vi "Migrate Measurements.vi"() -> ()   [LabVIEW 2021]
uses:
  _Measurement Migrator/Migrator/Queue Driver/controls/Queue Operations.ctl
  _Measurement Migrator/Migrator/Migration Logic/controls/Multiple Migration/Multiple Migration Data Holder.ctl
  <vilib>/Utility/sysdir.llb/System Directory Type.ctl
  <vilib>/Utility/miscctls.llb/LVRowAndColumnUnsignedTypeDef.ctl
  <vilib>/Utility/miscctls.llb/LVRowAndColumnTypeDef.ctl
  _Measurement Migrator/Migrator/Migrator Reusables/controls/Dictionary States.ctl
  <vilib>/Utility/cursorutil.llb/Set Cursor (Icon Pict).vi
  _Measurement Migrator/Migrator/Queue Driver/Queue Driver.lvlib
  _Measurement Migrator/Migrator/Migration Logic/Migrator.lvlib
  _Measurement Migrator/Migrator/Path Functions/Path Functions.lvlib
  _Measurement Migrator/Migrator/Multiple Migrator/Multiple Migrator.lvlib
  _Measurement Migrator/Migrator/Migrator Reusables/Migrator Reusables.lvlib
panel:
  out "error out":errorcluster
  in  "Tab Control":T1(tab)
  in  "Info":string
  in  "Select Measurement":path
  out "Warning":bool=TRUE caption="Warning:\nMeasurement should be an existing VI or folder path"
  in  "Populate measurements":bool
  in  "Select Project":path
  in  "Select all":bool
  in  "Back to Home":bool
  in  "List Plug-ins":bool
  in  "Select Measurements":string(tree)
  out "Selection warning":string="Atleast one measurement should be selected"
  out "Plug-in info":string="* Rename the Plug-in if required"
  out "Plug-in warning":string="Warning:\n1. Measurement plug-in name must be unique \n2. Plugin name cannot contain any of the following characters:\n         \\ / : * ? \" < > |"
  in  "Start Migration":bool
  in  "Back to Select":bool
  in  "List of Selected Measurements":i32(listbox)
  in  "Measurement Count":i32(slide)=6 caption="Migrating 1 of 1 measurement(s)" scale=0.0..100.0
  in  "Progress":i32(slide)=9 caption="Saving the project files..." scale=0.0..15.0
  in  "Review":bool
  in  "Migration Status":i32(listbox)
  in  "Back to Status":bool
  in  "Select Plug-in":string(combo) caption="Select Measurement plug-in to review"
  in  "Start Next":bool
  out "Launch Type Spec":string
  out "Launch Logic":string
  out "Launch UI":string
  # "* Project in which the measurement plug-in will be created"
  # "* Select a measurement vi or a folder containing measurements"
  # ".lvproj"
  # "Select the measurements to migrate"
  # "Review the Measurement:\n1. Review the Measurement UI. Click here to launch.\n2. Review the Measurement Logic VI. Click here to launch.\n3. Review the Type Specialization VI. Click here to launch."
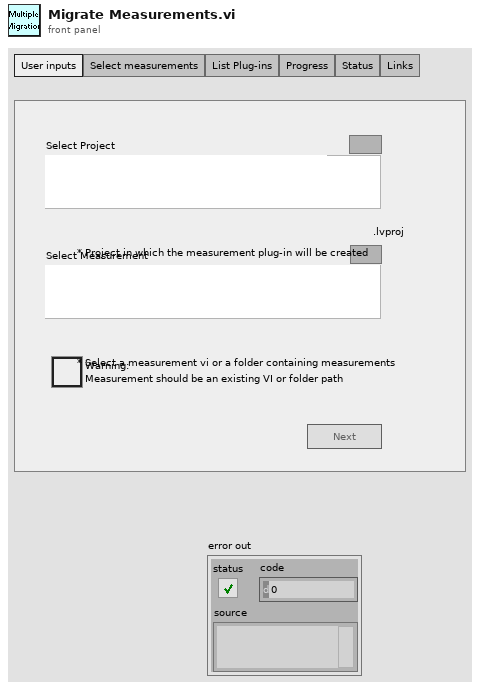
[diagram p1: front panel]
types:
  T1 = enum32{"User inputs", "Select measurements", "List Plug-ins", "Progress", "Status", "Links"}
  T2 = typedef "Queue Driver.lvlib/Queue Operations.ctl" = enum16{"Create Q", "Enqueue", "Enqueue N", "Dequeue", "Flush", "Release"}
  T3 = typedef "Migrator.lvlib/Multiple Migration Data Holder.ctl" = cluster{"Tree Reference":refnum<vi>, "LabVIEW Version":string, "Project path":path, "Create new project?":bool, "Measurement file/folder path":path, "Measurement folder selected?":bool, "Project warning":string, "Measurement warning":string, "Next clicked?":bool, "Measurement path changed?":bool, "Select all":bool, "Measurement folder Tags":string[], "Measurement file Tags":string[], "Selected cell Tag":string, "Measurement Plug-ins":string[][], "Measurement File Paths":path[], "Plugin Migration Value":i32, "Migration Count":i32, "Instrument containing subVIs":path[][], "Progress per measurement":i32, "Measurement Progress":i32, "Migration Status":string[][]}
  T4 = enum8{"Enabled", "Disabled", "Disabled and Grayed Out"}
  T5 = typedef "LVRowAndColumnUnsignedTypeDef.ctl" = cluster{"Row":u32, "Column":u32}
  T6 = typedef "LVRowAndColumnTypeDef.ctl" = cluster{"Row":i32, "Column":i32}
  T7 = typedef "Migrator Reusables.lvlib/Dictionary States.ctl" = enum16{"Set", "Get", "Delete", "Delete All"}
  T8 = typedef "System Directory Type.ctl" = i32
  T9 = typedef "LVPoint32TypeDef.ctl" = cluster{"Horizontal":i32, "Vertical":i32}
  T10 = typedef "Migrator.lvlib/Tree Items.ctl" = cluster{"Item name":string, "Indent":i32, "Tag":string}
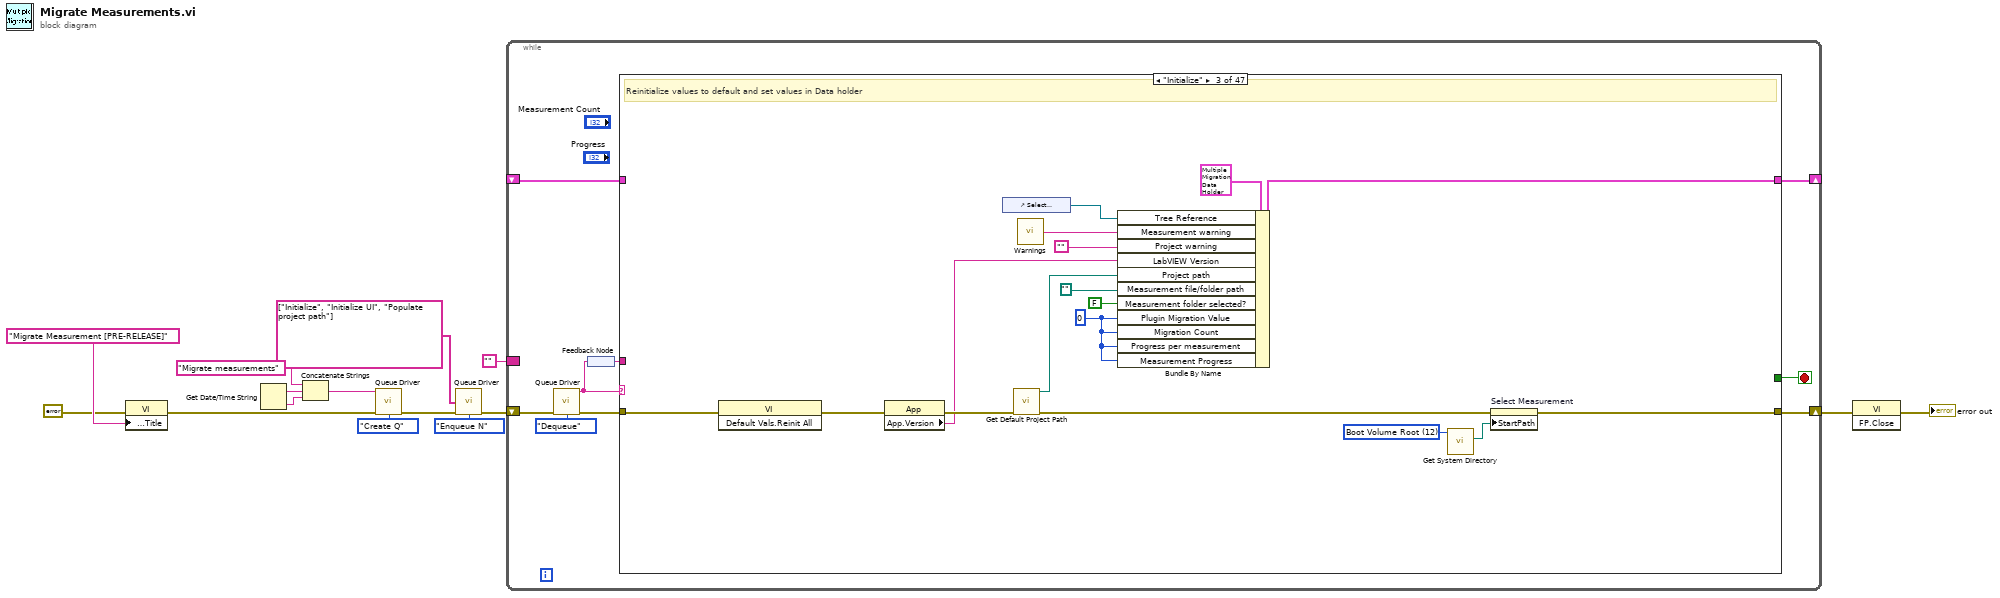
[diagram p0: block diagram]
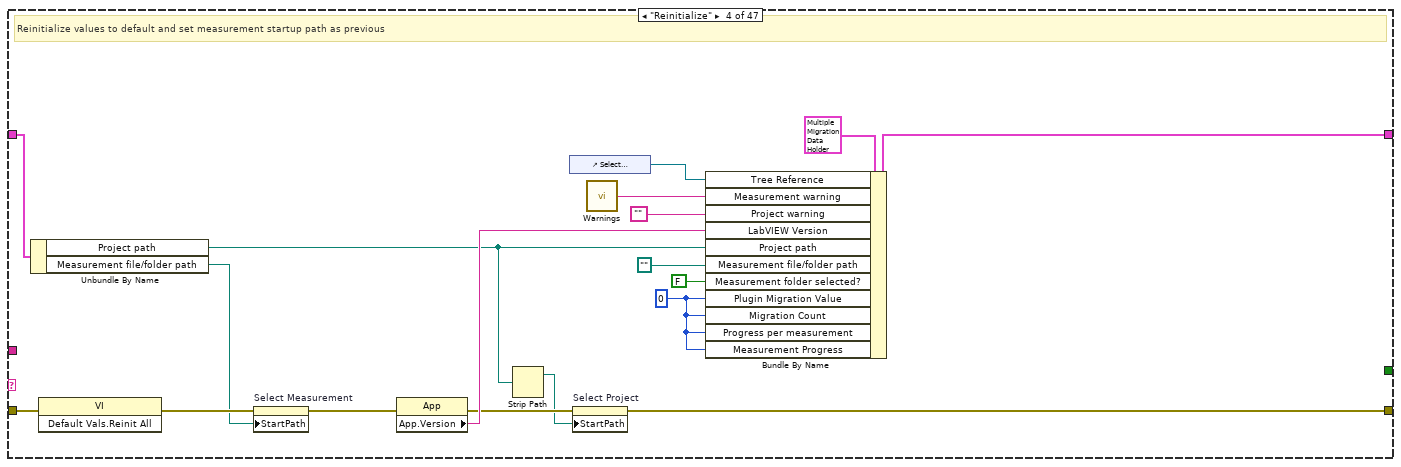
[diagram p4: hidden frame]
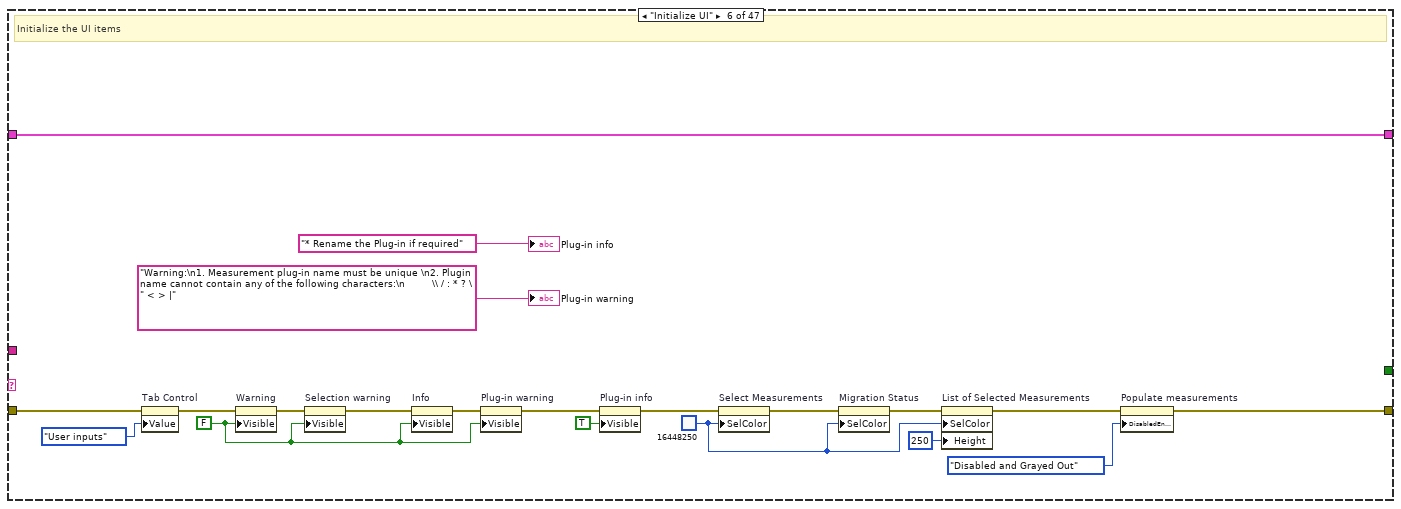
[diagram p6: hidden frame]
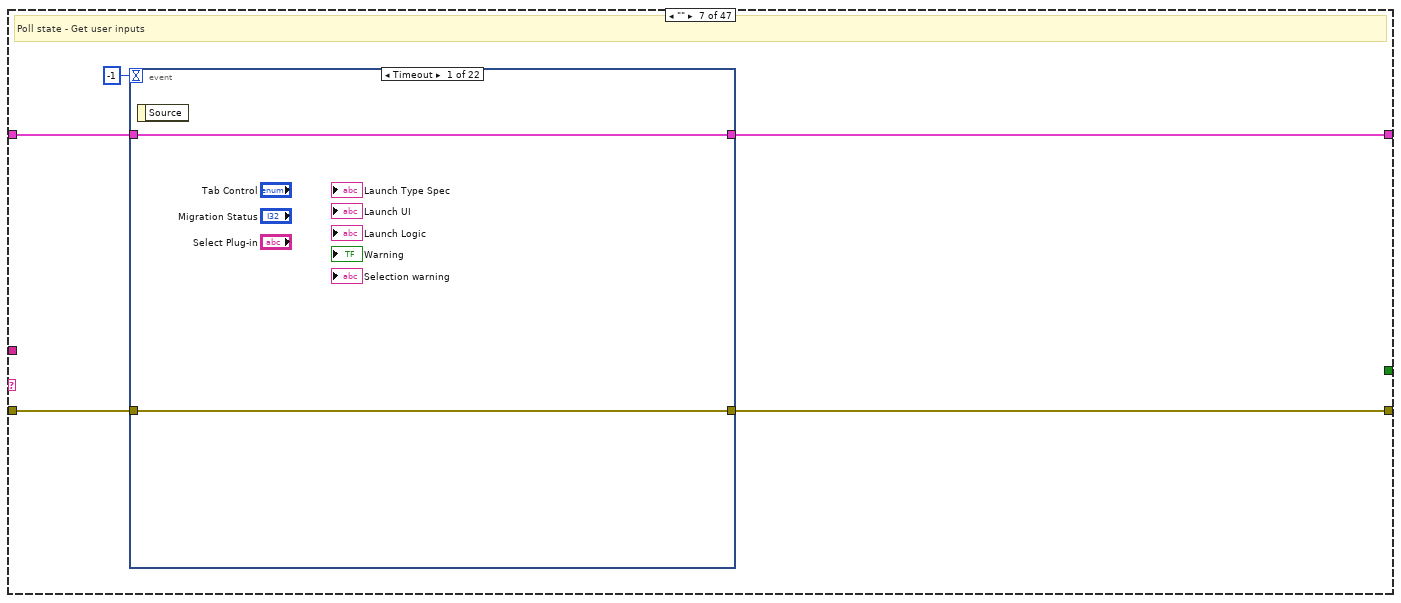
[diagram p7: hidden frame]
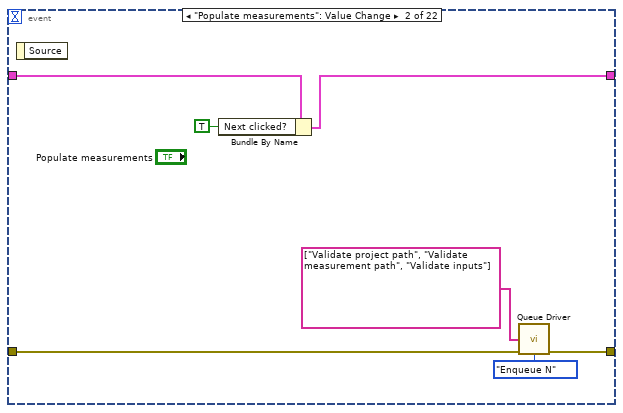
[diagram p8: hidden frame]
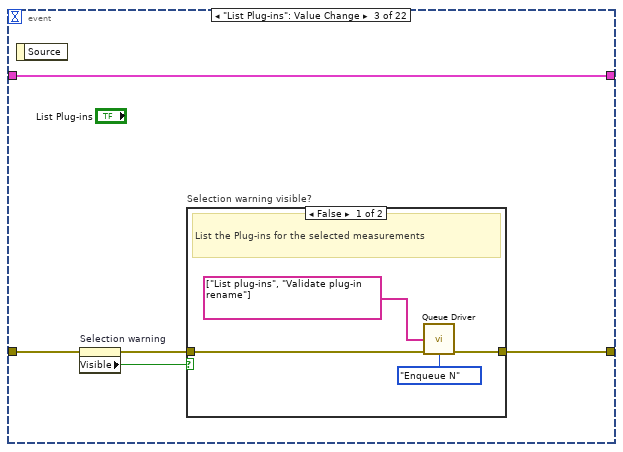
[diagram p9: hidden frame]
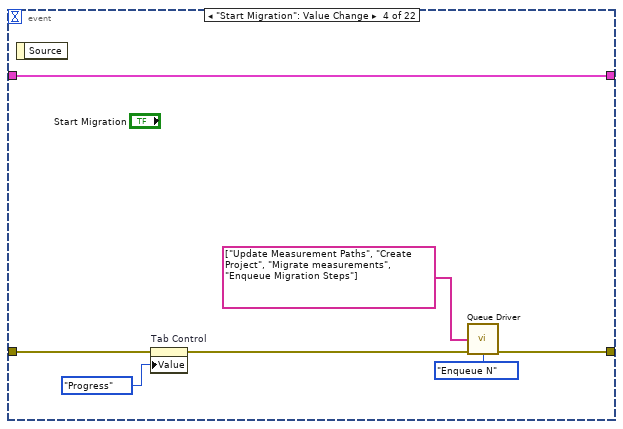
[diagram p11: hidden frame]
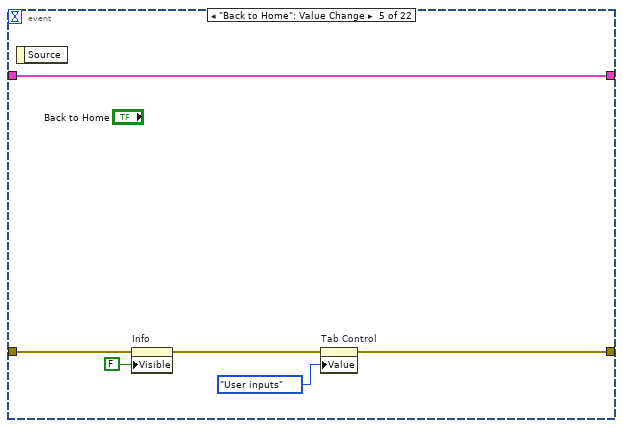
[diagram p12: hidden frame]
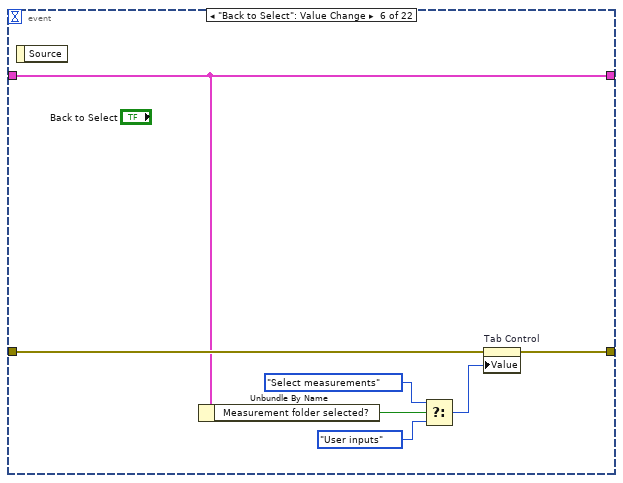
[diagram p13: hidden frame]
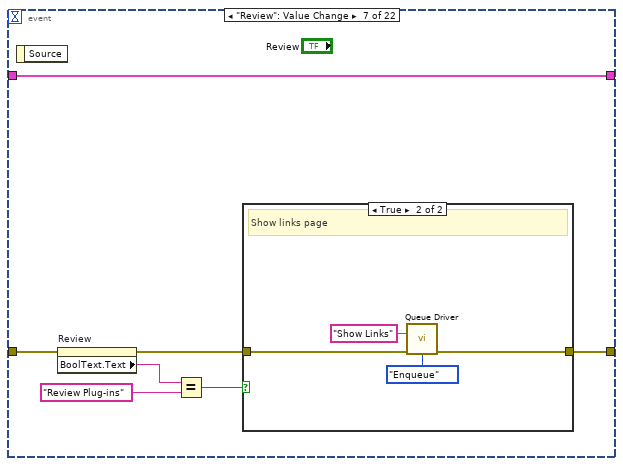
[diagram p14: hidden frame]
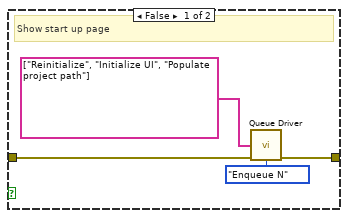
[diagram p15: hidden frame]
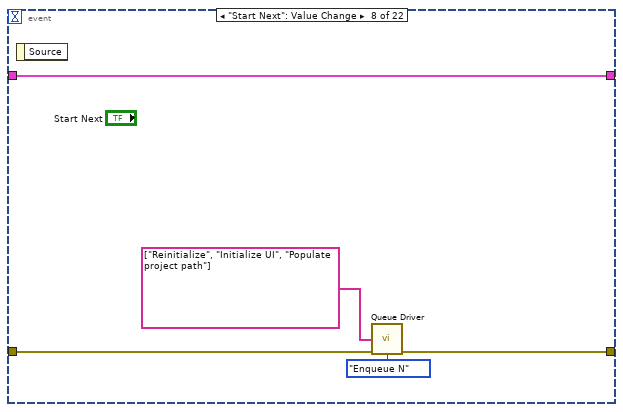
[diagram p16: hidden frame]
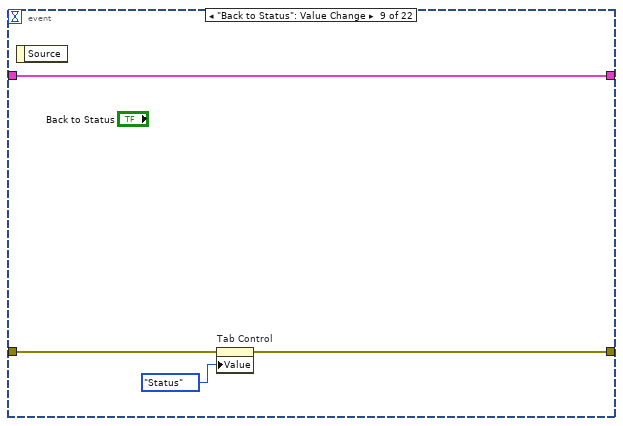
[diagram p17: hidden frame]
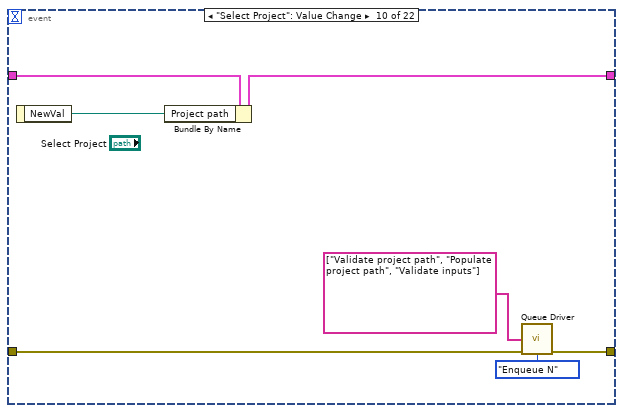
[diagram p18: hidden frame]
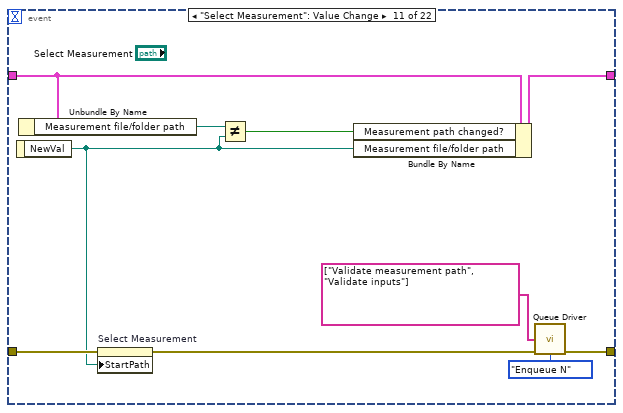
[diagram p19: hidden frame]
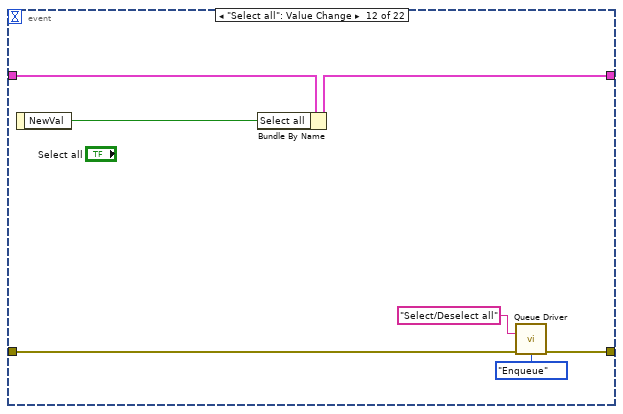
[diagram p20: hidden frame]
diagram:
  n1 = property class="VI"(error in=errorcluster {"status"=FALSE, "code"=0, "source"=""} ("error in (no error)"), "Front Panel.Title"="Migrate Measurement [PRE-RELEASE]" ("Front Panel Window:Title")) -> (error out=w1:errorcluster)  [unwired: 1 in, 1 out]
  n2 = Get Date/Time String() -> (date string=w12:string, time string=w11:string)  [unwired: 3 in]
  n3 = Concatenate Strings("Migrate measurements" ("string"), w12, w11) -> (w7:string)
  n4 = call "Queue Driver.vi"("Name"=w7, "error in (no error)"=w1, "Q Operations"=Queue_Operations."Create Q") -> ("error out"=w15:errorcluster)  [unwired: 11 in, 1 out]
  n5 = call "Queue Driver.vi"("States[]"=string[] ["Initialize", "Initialize UI", "Populate project path"], "error in (no error)"=w15, "Q Operations"=Queue_Operations."Enqueue N") -> ("error out"=w10:errorcluster)  [unwired: 11 in, 1 out]
  n6 = while {
    shift-right: [w23] -> w6
    shift-left: w10 -> [w24]
    shift-right: [w20] -> _
    shift-left: _ -> [w19]
    border: "" -> [_]
    stop <- w18 stop-if-true
    n7 = call "Queue Driver.vi"("error in (no error)"=w24, "Q Operations"=Queue_Operations."Dequeue") -> ("Dequeued State"=w17:string, "error out"=w22:errorcluster)  [unwired: 12 in]
    n8 = feedback #1() -> (w16:string)
    n9 = feedback-in #1(w17) -> ()
    n10 = case shown="\"Initialize\"" w17 {
      tunnel: w22 -> [w25 w28 w45 w63 w65 w85 w90 w262 w274 w285 w304 w328 w373 w390 w443 w468 w487 w544 w554 w560 w583 w593 w612 w629 w651 w658 w664 w670 w676 w682 w688 w694 w700 w706 w712 w718 w724 w730 w736 w758 w779 w791 w833 w842 w851 w872 w884]
      tunnel: [w25 w28 w34 w48 w65 w76 w89 w264 w274 w277 w303 w327 w373 w385 w431 w451 w474 w534 w554 w555 w580 w596 w611 w628 w650 w660 w666 w672 w678 w684 w690 w696 w702 w708 w714 w720 w726 w731 w740 w762 w779 w790 w830 w842 w848 w872 w874] -> w23
      tunnel: [w26 w27 w44 w62 w64 w81 w86 w263 w275 w280 w297 w315 w374 w391 w434 w466 w471 w539 w553 w575 w591 w605 w615 w648 w656 w662 w668 w674 w680 w686 w692 w698 w704 w710 w716 w722 w728 w734 w741 w763 w780 w795 w832 w843 w853 w873 w882] -> w20
      tunnel: w19 -> [w26 w27 _ w51 w64 w81 w87 w263 w275 w281 w299 w326 w374 w392 w435 w467 w472 w540 w553 w576 w591 w604 w615 w648 w656 w662 w668 w674 w680 w686 w692 w698 w704 w710 w716 w722 w728 w734 w742 w764 w780 w796 w832 w843 w853 w873 w882]
      tunnel: [_ _ _ _ _ _ _ _ _ _ _ _ _ _ _ _ _ _ _ _ _ _ _ _ _ _ _ _ _ _ _ _ _ _ _ _ _ _ _ _ _ _ _ _ _ _ TRUE] -> w18
      tunnel: w16 -> [_ _ _ _ _ _ _ _ _ _ _ _ _ _ _ _ _ _ _ _ _ _ _ _ _ _ _ _ _ _ _ _ _ _ _ _ _ _ _ _ _ _ _ _ w844 _ _]
      frame Default {
        # "Default case"
      }
      frame "/**********INITIALIZE**********/" {
      }
      frame "Initialize" {
        w29 = 0 ("Plugin Migration Value")
        w33 = T8 12 items=["User Home"=0, "User Desktop"=1, "User Documents"=2, "User Application Data"=3, "User Preferences"=4, "User Temporary"=5, "Public Documents"=6, "Public Application Data"=7, "Public Preferences"=8, "Public Cache"=13, "System Core Libraries"=9, "System Installed Libraries"=10, "Application Files"=11, "Boot Volume Root"=12] ("system directory type")
        # "Reinitialize values to default and set values in Data holder"
        n11 = invoke class="VI" method="Default Vals.Reinit All"(error in=w45) -> (error out=w42:errorcluster)  [unwired: 2 in, 2 out]
        n12 = property class="App"(error in=w42) -> (error out=w41:errorcluster, "App.Version"=w40:string)  [unwired: 1 in, 1 out]
        n13 = control-ref of="Select Measurements"() -> (w37:refnum<vi>)
        n14 = call "Get Default Project Path.vi"("error in"=w41) -> ("Project Path"=w43:path, "error out"=w35:errorcluster)  [unwired: 13 in]
        n15 = call "Warnings.vi"() -> ("Invalid measurement path"=w36:string)  [unwired: 8 in, 7 out]
        n16 = Bundle By Name(cluster=T3 {"Tree Reference"=refnum, "LabVIEW Version"="", "Project path"=path "", "Create new project?"=FALSE, "Measurement file/folder path"=path "", "Measurement folder selected?"=FALSE, "Project warning"="", "Measurement warning"="", "Next clicked?"=FALSE, "Measurement path changed?"=FALSE, "Select all"=FALSE, "Measurement folder Tags"=[], "Measurement file Tags"=[], "Selected cell Tag"="", "Measurement Plug-ins"=[], "Measurement File Paths"=[], "Plugin Migration Value"=0, "Migration Count"=0, "Instrument containing subVIs"=[], "Progress per measurement"=0, "Measurement Progress"=0, "Migration Status"=[]}, "Tree Reference"=w37, "Measurement warning"=w36, "Project warning"="", "LabVIEW Version"=w40, "Project path"=w43, "Measurement file/folder path"=path "", "Measurement folder selected?"=FALSE, "Plugin Migration Value"=w29, "Migration Count"=w29, "Progress per measurement"=w29, "Measurement Progress"=w29) -> (w44:T3)
        n17 = call <vilib>:"Get System Directory.vi"("system directory type"=w33) -> ("system directory"=w32:path)  [unwired: 10 in]
        n18 = property on="Select Measurement" class="Path"(error in=w35, "StartPath"=w32) -> (error out=w34:errorcluster)  [unwired: 1 in, 1 out]
      }
      frame "Reinitialize" {
        w54 = 0 ("Plugin Migration Value")
        # "Reinitialize values to default and set measurement startup path as previous"
        n19 = Unbundle By Name(w51) -> ("Project path"=w47:path, "Measurement file/folder path"=w50:path)
        n20 = invoke class="VI" method="Default Vals.Reinit All"(error in=w63) -> (error out=w53:errorcluster)  [unwired: 2 in, 2 out]
        n21 = property on="Select Measurement" class="Path"(error in=w53, "StartPath"=w50) -> (error out=w52:errorcluster)  [unwired: 1 in, 1 out]
        n22 = property class="App"(error in=w52) -> (error out=w49:errorcluster, "App.Version"=w61:string)  [unwired: 1 in, 1 out]
        n23 = Strip Path(path=w47) -> (stripped path=w46:path)  [unwired: 1 out]
        n24 = control-ref of="Select Measurements"() -> (w58:refnum<vi>)
        n25 = property on="Select Project" class="Path"(error in=w49, "StartPath"=w46) -> (error out=w48:errorcluster)  [unwired: 1 in, 1 out]
        n26 = call "Warnings.vi"() -> ("Invalid measurement path"=w57:string)  [unwired: 8 in, 7 out]
        n27 = Bundle By Name(cluster=T3 {"Tree Reference"=refnum, "LabVIEW Version"="", "Project path"=path "", "Create new project?"=FALSE, "Measurement file/folder path"=path "", "Measurement folder selected?"=FALSE, "Project warning"="", "Measurement warning"="", "Next clicked?"=FALSE, "Measurement path changed?"=FALSE, "Select all"=FALSE, "Measurement folder Tags"=[], "Measurement file Tags"=[], "Selected cell Tag"="", "Measurement Plug-ins"=[], "Measurement File Paths"=[], "Plugin Migration Value"=0, "Migration Count"=0, "Instrument containing subVIs"=[], "Progress per measurement"=0, "Measurement Progress"=0, "Migration Status"=[]}, "Tree Reference"=w58, "Measurement warning"=w57, "Project warning"="", "LabVIEW Version"=w61, "Project path"=w47, "Measurement file/folder path"=path "", "Measurement folder selected?"=FALSE, "Plugin Migration Value"=w54, "Migration Count"=w54, "Progress per measurement"=w54, "Measurement Progress"=w54) -> (w62:T3)
      }
      frame "/**********FP RELATED**********/" {
      }
      frame "Initialize UI" {
        w70 = FALSE ("Visible")
        w78 = u32 16448250 ("Selection Color")
        # "Initialize the UI items"
        n28 = property on="Tab Control" class="TabCtl (strict)"(error in=w85, "Value"=T1."User inputs" ("Tab Control")) -> (error out=w80:errorcluster)  [unwired: 1 in, 1 out]
        n29 = property on="Warning" class="Bool"(error in=w80, "Visible"=w70) -> (error out=w79:errorcluster)  [unwired: 1 in, 1 out]
        n30 = property on="Selection warning" class="Str"(error in=w79, "Visible"=w70) -> (error out=w74:errorcluster)  [unwired: 1 in, 1 out]
        n31 = property on="Info" class="Str"(error in=w74, "Visible"=w70) -> (error out=w73:errorcluster)  [unwired: 1 in, 1 out]
        n32 = property on="Plug-in warning" class="Str"(error in=w73, "Visible"=w70) -> (error out=w69:errorcluster)  [unwired: 1 in, 1 out]
        n33 = property on="Plug-in info" class="Str"(error in=w69, "Visible"=TRUE) -> (error out=w68:errorcluster)  [unwired: 1 in, 1 out]
        n34 = property on="Select Measurements" class="Tree (strict)"(error in=w68, "SelColor"=w78) -> (error out=w83:errorcluster)  [unwired: 1 in, 1 out]
        n35 = property on="Migration Status" class="MCListbox (strict)"(error in=w83, "SelColor"=w78) -> (error out=w82:errorcluster)  [unwired: 1 in, 1 out]
        n36 = property on="List of Selected Measurements" class="MCListbox (strict)"(error in=w82, "SelColor"=w78, "Height"=u32 250 ("Size:Height")) -> (error out=w77:errorcluster)  [unwired: 1 in, 1 out]
        n37 = property on="Populate measurements" class="Bool"(error in=w77, "DisabledEnum"=T4."Disabled and Grayed Out" ("Disabled")) -> (error out=w76:errorcluster)  [unwired: 1 in, 1 out]
        "Plug-in warning" <- "Warning:\n1. Measurement plug-in name must be unique \n2. Plugin name cannot contain any of the following characters:\n         \\ / : * ? \" < > |" ("f")
        "Plug-in info" <- "* Rename the Plug-in if required" ("Plug-in warning")
      }
      frame "" {
        # "Poll state - Get user inputs"
        n38 = event shown="[0] Timeout" {
          selector: _ -> [_ _ _ _ _ _ _ _ _ _ _ _ _ _ _ _ _ _ _ _ _ _]
          dyn-events: _ -> [_ _ _ _ _ _ _ _ _ _ _ _ _ _ _ _ _ _ _ _ _ _]
          timeout: -1 -> [_ _ _ _ _ _ _ _ _ _ _ _ _ _ _ _ _ _ _ _ _ _]
          tunnel: w90 -> [w92 w99 w102 w116 w119 w129 w133 w146 w153 w160 w166 w174 w185 w194 w202 w209 w212 w216 w222 w232 w244 w256]
          tunnel: [w92 w98 w103 w112 w122 w128 w135 w147 w152 w159 w169 w173 w180 w193 w200 w210 w213 w217 w224 w235 w246 w255] -> w89
          tunnel: w87 -> [w91 w95 w104 w113 w120 w127 w136 w149 w150 w157 w164 w177 w184 w195 w203 w211 w215 w219 w225 w236 w247 w257]
          tunnel: [w91 w94 w104 w113 w120 w127 w136 w149 w150 w156 w170 w176 w183 w195 w203 w211 w215 w219 w225 w236 w247 w257] -> w86
          event Timeout {
            # "Timeout"
            n39 = event-data() -> ()  [unwired: 1 in, 1 out]
          }
          event "Populate measurements": Value Change {
            n40 = event-data() -> ()  [unwired: 1 in, 1 out]
            n41 = Bundle By Name(cluster=w95, "Next clicked?"=TRUE) -> (w94:T3)
            n42 = call "Queue Driver.vi"("States[]"=string[] ["Validate project path", "Validate measurement path", "Validate inputs"], "error in (no error)"=w99, "Q Operations"=Queue_Operations."Enqueue N") -> ("error out"=w98:errorcluster)  [unwired: 11 in, 1 out]
          }
          event "List Plug-ins": Value Change {
            n43 = event-data() -> ()  [unwired: 1 in, 1 out]
            n44 = property on="Selection warning" class="Str"(error in=w102) -> (error out=w101:errorcluster, "Visible"=w100:bool)  [unwired: 1 in, 1 out]
            n45 = case "Selection warning visible?" shown="False" w100 {
              tunnel: w101 -> [w108 w109]
              tunnel: [w107 w109] -> w103
              frame False {
                # "List the Plug-ins for the selected measurements"
                n46 = call "Queue Driver.vi"("States[]"=string[] ["List plug-ins", "Validate plug-in rename"], "error in (no error)"=w108, "Q Operations"=Queue_Operations."Enqueue N") -> ("error out"=w107:errorcluster)  [unwired: 11 in, 1 out]
              }
              frame True {
                # "Pass"
              }
            }
          }
          event "Start Migration": Value Change {
            n47 = event-data() -> ()  [unwired: 1 in, 1 out]
            n48 = property on="Tab Control" class="TabCtl (strict)"(error in=w116, "Value"=T1."Progress" ("Tab Control")) -> (error out=w115:errorcluster)  [unwired: 1 in, 1 out]
            n49 = call "Queue Driver.vi"("States[]"=string[] ["Update Measurement Paths", "Create Project", "Migrate measurements", "Enqueue Migration Steps"], "error in (no error)"=w115, "Q Operations"=Queue_Operations."Enqueue N") -> ("error out"=w112:errorcluster)  [unwired: 11 in, 1 out]
          }
          event "Back to Home": Value Change {
            n50 = event-data() -> ()  [unwired: 1 in, 1 out]
            n51 = property on="Info" class="Str"(error in=w119, "Visible"=FALSE) -> (error out=w118:errorcluster)  [unwired: 1 in, 1 out]
            n52 = property on="Tab Control" class="TabCtl (strict)"(error in=w118, "Value"=T1."User inputs" ("Tab Control")) -> (error out=w122:errorcluster)  [unwired: 1 in, 1 out]
          }
          event "Back to Select": Value Change {
            n53 = event-data() -> ()  [unwired: 1 in, 1 out]
            n54 = Unbundle By Name(w127) -> ("Measurement folder selected?"=w126:bool)
            n55 = Select(t=T1."Select measurements" ("Tab Control"), s=w126, f=T1."User inputs" ("Tab Control")) -> (s? t:f=w123:T1)
            n56 = property on="Tab Control" class="TabCtl (strict)"(error in=w129, "Value"=w123) -> (error out=w128:errorcluster)  [unwired: 1 in, 1 out]
          }
          event "Review": Value Change {
            n57 = event-data() -> ()  [unwired: 1 in, 1 out]
            n58 = property on="Review" class="Bool"(error in=w133) -> (error out=w134:errorcluster, "BoolText.Text"=w132:string)  [unwired: 1 in, 1 out]
            n59 = Equal?(x=w132, y="Review Plug-ins") -> (x = y?=w130:bool)
            n60 = case shown="True" w130 {
              tunnel: [w138 w144] -> w135
              tunnel: w134 -> [w137 w141]
              frame False {
                # "Show start up page"
                n61 = call "Queue Driver.vi"("States[]"=string[] ["Reinitialize", "Initialize UI", "Populate project path"], "error in (no error)"=w137, "Q Operations"=Queue_Operations."Enqueue N") -> ("error out"=w138:errorcluster)  [unwired: 11 in, 1 out]
              }
              frame True {
                # "Show links page"
                n62 = call "Queue Driver.vi"("State"="Show Links", "error in (no error)"=w141, "Q Operations"=Queue_Operations."Enqueue") -> ("error out"=w144:errorcluster)  [unwired: 11 in, 1 out]
              }
            }
          }
          event "Start Next": Value Change {
            n63 = event-data() -> ()  [unwired: 1 in, 1 out]
            n64 = call "Queue Driver.vi"("States[]"=string[] ["Reinitialize", "Initialize UI", "Populate project path"], "error in (no error)"=w146, "Q Operations"=Queue_Operations."Enqueue N") -> ("error out"=w147:errorcluster)  [unwired: 11 in, 1 out]
          }
          event "Back to Status": Value Change {
            n65 = event-data() -> ()  [unwired: 1 in, 1 out]
            n66 = property on="Tab Control" class="TabCtl (strict)"(error in=w153, "Value"=T1."Status" ("Tab Control")) -> (error out=w152:errorcluster)  [unwired: 1 in, 1 out]
          }
          event "Select Project": Value Change {
            n67 = event-data() -> ("NewVal"=w155:path)  [unwired: 1 in]
            n68 = Bundle By Name(cluster=w157, "Project path"=w155) -> (w156:T3)
            n69 = call "Queue Driver.vi"("States[]"=string[] ["Validate project path", "Populate project path", "Validate inputs"], "error in (no error)"=w160, "Q Operations"=Queue_Operations."Enqueue N") -> ("error out"=w159:errorcluster)  [unwired: 11 in, 1 out]
          }
          event "Select Measurement": Value Change {
            n70 = event-data() -> ("NewVal"=w161:path)  [unwired: 1 in]
            n71 = Unbundle By Name(w164) -> ("Measurement file/folder path"=w162:path)
            n72 = property on="Select Measurement" class="Path"(error in=w166, "StartPath"=w161) -> (error out=w165:errorcluster)  [unwired: 1 in, 1 out]
            n73 = Not Equal?(x=w162, y=w161) -> (x != y?=w163:bool)
            n74 = Bundle By Name(cluster=w164, "Measurement path changed?"=w163, "Measurement file/folder path"=w161) -> (w170:T3)
            n75 = call "Queue Driver.vi"("States[]"=string[] ["Validate measurement path", "Validate inputs"], "error in (no error)"=w165, "Q Operations"=Queue_Operations."Enqueue N") -> ("error out"=w169:errorcluster)  [unwired: 11 in, 1 out]
          }
          event "Select all": Value Change {
            n76 = event-data() -> ("NewVal"=w175:bool)  [unwired: 1 in]
            n77 = Bundle By Name(cluster=w177, "Select all"=w175) -> (w176:T3)
            n78 = call "Queue Driver.vi"("State"="Select/Deselect all", "error in (no error)"=w174, "Q Operations"=Queue_Operations."Enqueue") -> ("error out"=w173:errorcluster)  [unwired: 11 in, 1 out]
          }
          event "Select Measurements": Mouse Down {
            n79 = event-data() -> ("Coords"=w178:T9)  [unwired: 1 in]
            n80 = invoke on="Select Measurements" class="Tree (strict)" method="Point To Row Column"(error in=w185, "Point"=w178) -> (error out=w181:errorcluster, "Tag"=w182:string, "InGlyph"=w179:bool)  [unwired: 6 in, 5 out]
            n81 = case "In Symbol?" shown="True" w179 {
              tunnel: w181 -> [w186 w190]
              tunnel: [w186 w189] -> w180
              frame False {
                # "Pass"
              }
              frame True {
                # "Update the selection of measurements"
                n82 = call "Queue Driver.vi"("State"="Measurement selection" ("State 2"), "error in (no error)"=w190, "Q Operations"=Queue_Operations."Enqueue") -> ("error out"=w189:errorcluster)  [unwired: 11 in, 1 out]
              }
            }
            n83 = Bundle By Name(cluster=w184, "Selected cell Tag"=w182) -> (w183:T3)
          }
          event "List of Selected Measurements": Edit Cell {
            n84 = event-data() -> ()  [unwired: 1 in, 1 out]
            n85 = call "Queue Driver.vi"("State"="Validate plug-in rename", "error in (no error)"=w194, "Q Operations"=Queue_Operations."Enqueue") -> ("error out"=w193:errorcluster)  [unwired: 11 in, 1 out]
          }
          event "List of Selected Measurements": Mouse Down {
            n86 = event-data() -> ("Coords"=w199:T9)  [unwired: 1 in, 7 out]
            n87 = invoke on="List of Selected Measurements" class="MCListbox (strict)" method="Point To Row Column"(error in=w202, "Point"=w199) -> (error out=w201:errorcluster, "CellPosition"=w196:T6)  [unwired: 5 in, 5 out]
            n88 = Unbundle By Name(w196) -> ("Column"=w198:i32)
            n89 = Not Equal To 0?(x=w198) -> (x != 0?=w197:bool)
            n90 = case shown="False" w197 {
              tunnel: w201 -> [w204 w207]
              tunnel: [w204 w206] -> w200
              tunnel: w196 -> [_ w205]
              frame False {
              }
              frame True {
                n91 = property on="List of Selected Measurements" class="MCListbox (strict)"(error in=w207, "EditPos"=w205) -> (error out=w206:errorcluster)  [unwired: 1 in, 1 out]
              }
            }
          }
          event "Select Plug-in": Value Change {
            n92 = event-data() -> ("NewVal"=w208:string)  [unwired: 1 in]
            n93 = call "Set Measurement Name.vi"("Name"=w208, "error in (no error)"=w209) -> ("error out"=w210:errorcluster)  [unwired: 13 in]
          }
          event "Launch UI", "Launch Logic", "Launch Type Spec": Mouse Enter {
            n94 = event-data() -> ()  [unwired: 1 in, 1 out]
            n95 = call-poly <vilib>:"Set Cursor.vi"("error in (no error)"=w212, "icon"=u16 6) -> ("error out"=w213:errorcluster)  [unwired: 8 in, 1 out]
          }
          event "Launch UI", "Launch Logic", "Launch Type Spec": Mouse Leave {
            n96 = event-data() -> ()  [unwired: 1 in, 1 out]
            n97 = call-poly <vilib>:"Set Cursor.vi"("error in (no error)"=w216, "icon"=u16 0) -> ("error out"=w217:errorcluster)  [unwired: 8 in, 1 out]
          }
          event "Launch UI": Mouse Down {
            n98 = event-data() -> ()  [unwired: 1 in, 1 out]
            n99 = property on="Select Plug-in" class="CmbBox"(error in=w222) -> (error out=w223:errorcluster, "Value"=w221:string)  [unwired: 1 in, 1 out]
            n100 = Empty String/Path?(string/path=w221) -> (empty?=w220:bool)
            n101 = case shown="False" w220 {
              tunnel: [w228 w230] -> w224
              tunnel: w223 -> [w226 w230]
              frame False {
                n102 = call "Measurement Plugin Path.vi"("error in (no error)"=w226) -> ("Measurement UI"=w227:path, "error out"=w229:errorcluster)  [unwired: 2 in, 11 out]
                n103 = call "Open VI.vi"("Logic VI Path"=w227, "error in (no error)"=w229) -> ("error out"=w228:errorcluster)  [unwired: 13 in]
              }
              frame True {
              }
            }
          }
          event "Launch Logic": Mouse Down {
            n104 = event-data() -> ()  [unwired: 1 in, 1 out]
            n105 = property on="Select Plug-in" class="CmbBox"(error in=w232) -> (error out=w233:errorcluster, "Value"=w234:string)  [unwired: 1 in, 1 out]
            n106 = Empty String/Path?(string/path=w234) -> (empty?=w231:bool)
            n107 = case shown="False" w231 {
              tunnel: [w239 w241] -> w235
              tunnel: w233 -> [w238 w241]
              frame False {
                n108 = call "Measurement Plugin Path.vi"("error in (no error)"=w238) -> ("Logic VI Path"=w237:path, "error out"=w240:errorcluster)  [unwired: 2 in, 11 out]
                n109 = call "Open VI.vi"("Logic VI Path"=w237, "error in (no error)"=w240) -> ("error out"=w239:errorcluster)  [unwired: 13 in]
              }
              frame True {
              }
            }
          }
          event "Launch Type Spec": Mouse Down {
            n110 = event-data() -> ()  [unwired: 1 in, 1 out]
            n111 = property on="Select Plug-in" class="CmbBox"(error in=w244) -> (error out=w243:errorcluster, "Value"=w245:string)  [unwired: 1 in, 1 out]
            n112 = Empty String/Path?(string/path=w245) -> (empty?=w242:bool)
            n113 = case shown="False" w242 {
              tunnel: [w250 w252] -> w246
              tunnel: w243 -> [w249 w252]
              frame False {
                n114 = call "Measurement Plugin Path.vi"("error in (no error)"=w249) -> ("Type Specialization"=w248:path, "error out"=w251:errorcluster)  [unwired: 2 in, 11 out]
                n115 = call "Open VI.vi"("Logic VI Path"=w248, "error in (no error)"=w251) -> ("error out"=w250:errorcluster)  [unwired: 13 in]
              }
              frame True {
              }
            }
          }
          event Panel Close? {
            n116 = event-data() -> ()  [unwired: 1 in, 1 out]
            n117 = call "Queue Driver.vi"("State"="Exit", "error in (no error)"=w256, "Q Operations"=Queue_Operations."Enqueue") -> ("error out"=w255:errorcluster)  [unwired: 11 in, 1 out]
            n118 = event-data("Discard?"=TRUE) -> ()  [unwired: 1 in, 1 out]
          }
        }
      }
      frame "Populate project path" {
        # "Populate the validated project path in the control"
        n119 = Unbundle By Name(w263) -> ("Project warning"=w260:string, "Project path"=w261:path)
        n120 = Empty String/Path?(string/path=w260) -> (empty?=w259:bool)
        n121 = case "Valid project?" shown="True" w259 {
          tunnel: [w265 w273] -> w264
          tunnel: w262 -> [w265 w272]
          tunnel: w261 -> [_ w267]
          frame False {
            # "Pass"
          }
          frame True {
            # "Populate the path in the control"
            n122 = call <vilib>:"Get File Extension.vi"("error in (no error)"=w272, "file"=w267) -> ("error out"=w271:errorcluster, "filename without extension"=w270:string)  [unwired: 5 in, 3 out]
            n123 = Concatenate Strings("..\\" ("string"), w270) -> (w268:string)
            n124 = Build Path(base path=w267, name or relative path=w268) -> (appended path=w266:path)
            n125 = property on="Select Project" class="Path"(error in=w271, "Value"=w266) -> (error out=w273:errorcluster)  [unwired: 1 in, 1 out]
          }
        }
      }
      frame "/**********INPUT VALIDATION**********/" {
      }
      frame "Validate project path" {
        # "Validate the project path and set warning if required"
        n126 = Unbundle By Name(w281) -> ("Project path"=w282:path, "LabVIEW Version"=w283:string)
        n127 = call <vilib>:"Is Path and Not Empty.vi"("path"=w282) -> ("Is Path and Not Empty?"=w284:bool)  [unwired: 4 in]
        n128 = case "Is Path and not empty?" shown="True" w284 {
          tunnel: w285 -> [w288 w295]
          tunnel: [w288 w294] -> w277
          tunnel: [w286 w293] -> w276
          tunnel: w283 -> [_ w292]
          tunnel: w282 -> [w287 w291]
          tunnel: [_ w290] -> w279
          tunnel: [w287 w289] -> w278
          frame False {
            # "Set warning"
            n129 = call "Warnings.vi"() -> ("Invalid project path"=w286:string)  [unwired: 8 in, 7 out]
          }
          frame True {
            # "Validate the path"
            n130 = call "Validate Project Path.vi"("Project path in"=w291, "LabVIEW Version"=w292, "error in (no error)"=w295) -> ("Validated project path"=w289:path, "New project?"=w290:bool, "Warning"=w293:string, "error out"=w294:errorcluster)  [unwired: 9 in]
          }
        }
        n131 = Bundle By Name(cluster=w281, "Project path"=w278, "Create new project?"=w279, "Project warning"=w276) -> (w280:T3)
      }
      frame "Validate measurement path" {
        # "Validate the measurement path and set warning if required"
        n132 = Unbundle By Name(w299) -> ("Measurement file/folder path"=w301:path, "LabVIEW Version"=w302:string)
        n133 = call <vilib>:"Is Path and Not Empty.vi"("path"=w301) -> ("Is Path and Not Empty?"=w300:bool)  [unwired: 4 in]
        n134 = case "Is Path and not empty?" shown="True" w300 {
          tunnel: w304 -> [w306 w312]
          tunnel: w301 -> [_ w311]
          tunnel: w302 -> [_ w310]
          tunnel: [w306 w309] -> w303
          tunnel: [w305 w308] -> w296
          tunnel: [_ w307] -> w298
          frame False {
            # "Set warning"
            n135 = call "Warnings.vi"() -> ("Invalid measurement path"=w305:string)  [unwired: 8 in, 7 out]
          }
          frame True {
            # "Validate the path"
            n136 = call "Validate Measurement Path.vi"("Measurement path"=w311, "LabVIEW version"=w310, "error in (no error)"=w312) -> ("Folder?"=w307:bool, "Warning"=w308:string, "error out"=w309:errorcluster)  [unwired: 10 in]
          }
        }
        n137 = Bundle By Name(cluster=w299, "Measurement folder selected?"=w298, "Measurement warning"=w296) -> (w297:T3)
      }
      frame "Validate inputs" {
        # "Validate the project path and measurement path inputs"
        n138 = Unbundle By Name(w326) -> ("Project warning"=w320:string, "Measurement warning"=w325:string, "Next clicked?"=w321:bool, "Project warning"=w319:string, "Measurement warning"=w318:string, "Measurement folder selected?"=w317:bool, "Measurement path changed?"=w316:bool)
        n139 = Empty String/Path?(string/path=w325) -> (empty?=w324:bool)
        n140 = Empty String/Path?(string/path=w320) -> (empty?=w323:bool)
        n141 = And(x=w323, y=w324) -> (x .and. y?=w322:bool)
        n142 = case "Valid inputs?" shown="False" w322 {
          tunnel: w328 -> [w342 w352]
          tunnel: [w337 w348] -> w327
          tunnel: w321 -> [_ w346]
          tunnel: w319 -> [w330 _]
          tunnel: w318 -> [w333 _]
          tunnel: w317 -> [_ w345]
          tunnel: w316 -> [w329 w344]
          tunnel: [w329 w343] -> w313
          frame False {
            # "Set the appropriate warning"
            n143 = call "Edit Warning.vi"("Warning in"=w330) -> ("Warning out"=w332:string)  [unwired: 6 in]
            n144 = call "Edit Warning.vi"("Warning in"=w333) -> ("Warning out"=w331:string)  [unwired: 6 in]
            n145 = Concatenate Strings("Warning:" ("string"), "\n", w332, w331) -> (w335:string)
            n146 = call "Get Warning Position.vi"("Warning"=w335) -> ("Warning position"=w334:i32)  [unwired: 6 in]
            n147 = property on="Warning" class="Bool"(error in=w342, "Visible"=TRUE, "Caption.Text"=w335, "Caption.Top"=w334) -> (error out=w338:errorcluster)  [unwired: 1 in, 1 out]
            n148 = property on="Populate measurements" class="Bool"(error in=w338, "DisabledEnum"=T4."Disabled and Grayed Out" ("Disabled")) -> (error out=w337:errorcluster)  [unwired: 1 in, 1 out]
          }
          frame True {
            # "Check if next is clicked and make the warning invisible"
            n149 = case "Next clicked?" shown="True" w346 {
              tunnel: w352 -> [w354 w359]
              tunnel: [w354 w358] -> w351
              tunnel: w345 -> [_ w357]
              tunnel: w344 -> [w353 w356]
              tunnel: [w353 FALSE] -> w343
              frame False {
                # "Pass"
              }
              frame True {
                # "Populate measurements if folder is selected and List the plug-ins if not"
                n150 = case "Measurement path changed?" shown="True" w356 {
                  tunnel: w359 -> [w365 w372]
                  tunnel: [w364 w371] -> w358
                  tunnel: w357 -> [w360 w366]
                  frame False {
                    # "Measurement folder?"
                    n151 = Select(t=T1."Select measurements" ("Tab Control"), s=w360, f=T1."List Plug-ins" ("Tab Control")) -> (s? t:f=w361:T1)
                    n152 = property on="Tab Control" class="TabCtl (strict)"(error in=w365, "Value"=w361) -> (error out=w364:errorcluster)  [unwired: 1 in, 1 out]
                  }
                  frame True {
                    # "Measurement folder?"
                    n153 = Select(t="Populate measurements" ("State 2"), s=w366, f="List plug-ins" ("State 2")) -> (s? t:f=w367:string)
                    n154 = call "Queue Driver.vi"("State"=w367, "error in (no error)"=w372, "Q Operations"=Queue_Operations."Enqueue") -> ("error out"=w371:errorcluster)  [unwired: 11 in, 1 out]
                  }
                }
              }
            }
            n155 = property on="Warning" class="Bool"(error in=w351, "Visible"=FALSE) -> (error out=w349:errorcluster)  [unwired: 1 in, 1 out]
            n156 = property on="Populate measurements" class="Bool"(error in=w349, "DisabledEnum"=T4."Enabled" ("Disabled")) -> (error out=w348:errorcluster)  [unwired: 1 in, 1 out]
          }
        }
        n157 = Bundle By Name(cluster=w326, "Next clicked?"=FALSE, "Measurement path changed?"=w313) -> (w315:T3)
      }
      frame "/**********FUNCTIONALITY**********/" {
      }
      frame "Populate measurements" {
        w379 = TRUE ("Visible")
        # "Populate the measurements in the Tree and set icon to the items"
        n158 = Unbundle By Name(w392) -> ("Tree Reference"=w386:refnum<vi>, "Measurement file/folder path"=w395:path, "LabVIEW Version"=w393:string)
        n159 = call "Set Cursor Icon.vi"("Cursor icon"=u16 2, "error in (no error)"=w390) -> ("error out"=w389:errorcluster)  [unwired: 13 in]
        n160 = property on="Info" class="Str"(error in=w389, "Visible"=w379, "Text.FontBold"=w379, "Text.Text"="Populating the measurements..." ("Info")) -> (error out=w388:errorcluster)  [unwired: 1 in, 1 out]
        n161 = call "Get Measurements.vi"("Input path"=w395, "LabVIEW version"=w393, "error in (no error)"=w388) -> ("Error?"=w380:string, "VI list"=w382:T10[], "Folder list"=w381:T10[], "error out"=w394:errorcluster)  [unwired: 9 in]
        n162 = Empty String/Path?(string/path=w380) -> (empty?=w383:bool)
        n163 = case "No error occured during get measurements?" shown="True" w383 {
          tunnel: w394 -> [w396 w428]
          tunnel: w392 -> [w403 w427]
          tunnel: [w402 w426] -> w391
          tunnel: w386 -> [w401 w425]
          tunnel: [w399 w424] -> w376
          tunnel: w382 -> [_ w415]
          tunnel: w381 -> [_ w414]
          tunnel: w380 -> [w400 _]
          frame False {
            # "Update the warning"
            n164 = Bundle By Name(cluster=w403, "Tree Reference"=w401, "Measurement warning"=w400) -> (w402:T3)
            n165 = call "Queue Driver.vi"("State"="Validate inputs", "error in (no error)"=w396, "Q Operations"=Queue_Operations."Enqueue") -> ("error out"=w399:errorcluster)  [unwired: 11 in, 1 out]
          }
          frame True {
            w413 = FALSE
            # "Populate the Tree with the measurements"
            n166 = call "Populate Tree.vi"("TreeControl in"=w425, "VI list"=w415, "Folder list"=w414, "error in (no error)"=w428) -> ("TreeControl out"=w422:refnum<vi>, "error out"=w423:errorcluster)  [unwired: 10 in]
            n167 = call "Set Tree Item Icon.vi"("TreeControl in"=w422, "error in (no error)"=w423) -> ("TreeControl out"=w418:refnum<vi>, "Measurement folder Tags"=w416:string[], "Measurement file Tags"=w417:string[], "error out"=w421:errorcluster)  [unwired: 10 in]
            n168 = Empty Array?(array=w417) -> (empty?=w406:bool)
            n169 = Select(t="No Measurement found in the folder" ("Warning"), s=w406, f="Atleast one measurement should be selected" ("Text.Text")) -> (s? t:f=w407:string)
            n170 = property on="Selection warning" class="Str"(error in=w421, "Visible"=TRUE, "Text.Text"=w407) -> (error out=w412:errorcluster)  [unwired: 1 in, 1 out]
            n171 = Select(t=T4."Disabled and Grayed Out" ("Disabled"), s=w406, f=T4."Enabled") -> (s? t:f=w405:T4)
            n172 = Bundle By Name(cluster=w427, "Tree Reference"=w418, "Measurement folder Tags"=w416, "Measurement file Tags"=w417, "Select all"=w413) -> (w426:T3)
            n173 = property on="Select all" class="Bool (strict)"(error in=w412, "Value"=w413, "DisabledEnum"=w405) -> (error out=w419:errorcluster)  [unwired: 1 in, 1 out]
            n174 = property on="Tab Control" class="TabCtl (strict)"(error in=w419, "Value"=T1."Select measurements" ("Tab Control")) -> (error out=w424:errorcluster)  [unwired: 1 in, 1 out]
          }
        }
        n175 = property on="Info" class="Str"(error in=w376, "Visible"=FALSE) -> (error out=w375:errorcluster)  [unwired: 1 in, 1 out]
        n176 = call "Set Cursor Icon.vi"("Cursor icon"=u16 0, "error in (no error)"=w375) -> ("error out"=w385:errorcluster)  [unwired: 13 in]
      }
      frame "Select/Deselect all" {
        # "Update the selection of items in the Tree based on the value of Select all"
        n177 = call "Set Cursor Icon.vi"("Cursor icon"=u16 2, "error in (no error)"=w443) -> ("error out"=w432:errorcluster)  [unwired: 13 in]
        n178 = Unbundle By Name(w435) -> ("Tree Reference"=w436:refnum<vi>, "Measurement folder Tags"=w438:string[], "Measurement file Tags"=w440:string[], "Select all"=w442:bool)
        n179 = Not(x=w442) -> (.not. x?=w444:bool)
        n180 = call "Tree Icons.vi"() -> ("Not Selected"=w446:i32, "Selected"=w447:i32)  [unwired: 6 in]
        n181 = property on="Selection warning" class="Str"(error in=w432, "Text.Text"="Atleast one measurement should be selected", "Visible"=w444) -> (error out=w441:errorcluster)  [unwired: 1 in, 1 out]
        n182 = Select(t=w447, s=w442, f=w446) -> (s? t:f=w439:i32)
        n183 = call "Update Tree Item Icon.vi"("TreeControl in"=w436, "Measurement folder Tags"=w438, "Measurement file Tags"=w440, "Icon"=w439, "error in (no error)"=w441) -> ("TreeControl out"=w433:refnum<vi>, "error out"=w437:errorcluster)  [unwired: 9 in]
        n184 = Bundle By Name(cluster=w435, "Tree Reference"=w433) -> (w434:T3)
        n185 = call "Set Cursor Icon.vi"("Cursor icon"=u16 0, "error in (no error)"=w437) -> ("error out"=w431:errorcluster)  [unwired: 13 in]
      }
      frame "Measurement selection" {
        # "Update the icons of the Tree items based on the selection"
        n186 = call "Set Cursor Icon.vi"("Cursor icon"=u16 2, "error in (no error)"=w468) -> ("error out"=w453:errorcluster)  [unwired: 13 in]
        n187 = Unbundle By Name(w467) -> ("Tree Reference"=w448:refnum<vi>, "Measurement folder Tags"=w458:string[], "Measurement file Tags"=w457:string[], "Selected cell Tag"=w459:string)
        n188 = call "Update Tree Item Selection.vi"("TreeControl in"=w448, "Measurement folder Tags"=w458, "Measurement file Tags"=w457, "Selected cell Tag"=w459, "error in (no error)"=w453) -> ("TreeControl out"=w454:refnum<vi>, "error out"=w464:errorcluster)  [unwired: 9 in]
        n189 = Insert Into Array(array=w458, new element=w457) -> (w460:string[])  [unwired: 1 in]
        n190 = call "Verify Select All.vi"("TreeControl in"=w454, "Measurement Tags"=w460, "error in (no error)"=w464) -> ("TreeControl out"=w456:refnum<vi>, "Select"=w449:bool, "Deselect"=w455:bool, "error out"=w463:errorcluster)  [unwired: 9 in]
        n191 = Bundle By Name(cluster=w467, "Tree Reference"=w456, "Select all"=w449) -> (w466:T3)
        n192 = property on="Select all" class="Bool (strict)"(error in=w463, "Value"=w449) -> (error out=w462:errorcluster)  [unwired: 1 in, 1 out]
        n193 = property on="Selection warning" class="Str"(error in=w462, "Text.Text"="Atleast one measurement should be selected", "Visible"=w455) -> (error out=w465:errorcluster)  [unwired: 1 in, 1 out]
        n194 = call "Set Cursor Icon.vi"("Cursor icon"=u16 0, "error in (no error)"=w465) -> ("error out"=w451:errorcluster)  [unwired: 13 in]
      }
      frame "List plug-ins" {
        # "List the Plug-in names of the selected measurements"
        n195 = Unbundle By Name(w472) -> ("Tree Reference"=w477:refnum<vi>, "Measurement file Tags"=w483:string[], "Measurement folder selected?"=w486:bool, "Measurement file/folder path"=w485:path)
        n196 = call "Set Cursor Icon.vi"("Cursor icon"=u16 2, "error in (no error)"=w487) -> ("error out"=w476:errorcluster)  [unwired: 13 in]
        n197 = case "Measurement Folder?" shown="True" w486 {
          tunnel: w476 -> [w502 w508]
          tunnel: w485 -> [w501 _]
          tunnel: [w500 w505] -> w484
          tunnel: [w498 w504] -> w470
          tunnel: w483 -> [_ w507]
          tunnel: w477 -> [w497 w506]
          tunnel: [w497 w503] -> w469
          frame False {
            # "Get the plug-in name of the selected measurement file"
            n198 = call <vilib>:"Get File Extension.vi"("error in (no error)"=w502, "file"=w501) -> ("error out"=w500:errorcluster, "filename without extension"=w496:string)  [unwired: 5 in, 3 out]
            n199 = Build Array(w496, w496) -> (w499:string[])
            n200 = Build Array(w499) -> (w498:string[][])
          }
          frame True {
            # "Get the plug-in names of all the selected files in the measurement folder"
            n201 = call "Get Selected Measurements.vi"("Tree control in"=w506, "Measurement file Tags"=w507, "error in (no error)"=w508) -> ("Tree control out"=w503:refnum<vi>, "Measurement Plug-ins"=w504:string[][], "error out"=w505:errorcluster)  [unwired: 10 in]
          }
        }
        n202 = property on="List of Selected Measurements" class="MCListbox (strict)"(error in=w484, "ItemNames"=w470, "TopLeft"=T5 {"Row"=0, "Column"=0} ("Top Left Visible Cell")) -> (error out=w482:errorcluster)  [unwired: 1 in, 1 out]
        n203 = Bundle By Name(cluster=w472, "Tree Reference"=w469, "Measurement Plug-ins"=w470) -> (w471:T3)
        n204 = Array Size(array=w470) -> (size(s)=w480:i32[])
        n205 = Index Array(array=w480) -> (element=w479:i32)  [unwired: 1 in]
        n206 = for {
          N: w479 -> [_]
          shift-right: [w493] -> w481
          shift-left: w482 -> [w494]
          i -> [w490]
          # "Set the row size for the occupied rows"
          n207 = Bundle By Name(cluster=T6 {"Row"=0, "Column"=0} ("Active Cell:Active Cell"), "Row"=w490) -> (w492:T6)
          n208 = property on="List of Selected Measurements" class="MCListbox (strict)"(error in=w494, "ActiveCell"=w492, "Height"=u32 18 ("Active Cell:Cell Size:Height")) -> (error out=w493:errorcluster)  [unwired: 1 in, 1 out]
        }
        n209 = property on="Tab Control" class="TabCtl (strict)"(error in=w481, "Value"=T1."List Plug-ins" ("Tab Control")) -> (error out=w489:errorcluster)  [unwired: 1 in, 1 out]
        n210 = call "Set Cursor Icon.vi"("Cursor icon"=u16 0, "error in (no error)"=w489) -> ("error out"=w474:errorcluster)  [unwired: 13 in]
      }
      frame "Validate plug-in rename" {
        # "Validate the name of the Plug-in after rename"
        n211 = call "Set Cursor Icon.vi"("Cursor icon"=u16 2, "error in (no error)"=w544) -> ("error out"=w536:errorcluster)  [unwired: 13 in]
        n212 = property on="List of Selected Measurements" class="MCListbox (strict)"(error in=w536) -> (error out=w528:errorcluster, "ItemNames"=w542:string[][])  [unwired: 1 in, 1 out]
        n213 = Unbundle By Name(w540) -> ("Measurement Plug-ins"=w538:string[][], "Project path"=w526:path)
        n214 = Index Array(array=w542, index (col)=1 ("disabled index (col)")) -> (element=w511:string[])  [unwired: 1 in]
        n215 = call "Get Libraries in Project.vi"("Project path"=w526, "error in (no error)"=w528) -> ("Project exists?"=w525:bool, "Library names"=w524:string[], "error out"=w527:errorcluster)  [unwired: 11 in]
        n216 = Index Array(array=w538, index (col)=1 ("disabled index (col)")) -> (element=w510:string[])  [unwired: 1 in]
        n217 = for {
          shift-right: [w551] -> w521
          shift-left: w527 -> [w552]
          tunnel: w511 -> [w548] mode=indexing
          tunnel: w525 -> [w550]
          tunnel: w524 -> [w549]
          tunnel: [w546] -> w512 mode=indexing
          tunnel: w510 -> [w547] mode=indexing
          tunnel: [w545] -> w509 mode=indexing
          # "Validate the plug-in names"
          n218 = call "Validate Plugin Name.vi"("Project exists?"=w550, "Library names"=w549, "Plug-in name"=w548, "error in (no error)"=w552) -> ("Valid Name?"=w546:bool, "error out"=w551:errorcluster)  [unwired: 10 in]
          n219 = Swap Values(12:w547, 13:w546, 14:w548) -> (1:w545:string)  [unwired: 1 out]
        }
        n220 = call "Set Plug-in Name Warning.vi"("Valid Name?"=w512, "Validated names"=w509, "error in (no error)"=w521) -> ("Warning?"=w522:bool, "error out"=w520:errorcluster)  [unwired: 11 in]
        n221 = Replace Array Subset(array=w538, new element=w509, index (col)=1 ("disabled index (col)")) -> (w513:string[][])  [unwired: 1 in]
        n222 = property on="Plug-in warning" class="Str"(error in=w520, "Visible"=w522) -> (error out=w532:errorcluster)  [unwired: 1 in, 1 out]
        n223 = Swap Values(12:u32 250 ("Size:Height"), 13:w522, 14:210 ("x")) -> (1:w523:u32)  [unwired: 1 out]
        n224 = Bundle By Name(cluster=w540, "Measurement Plug-ins"=w513) -> (w539:T3)
        n225 = property on="List of Selected Measurements" class="MCListbox (strict)"(error in=w532, "ItemNames"=w513, "Height"=w523) -> (error out=w529:errorcluster)  [unwired: 1 in, 1 out]
        n226 = Not(x=w522) -> (.not. x?=w517:bool)
        n227 = property on="Plug-in info" class="Str"(error in=w529, "Visible"=w517) -> (error out=w519:errorcluster)  [unwired: 1 in, 1 out]
        n228 = Select(t=T4."Enabled", s=w517, f=T4."Disabled and Grayed Out" ("Disabled")) -> (s? t:f=w514:T4)
        n229 = property on="Start Migration" class="Bool"(error in=w519, "DisabledEnum"=w514) -> (error out=w518:errorcluster)  [unwired: 1 in, 1 out]
        n230 = call "Set Cursor Icon.vi"("Cursor icon"=u16 0, "error in (no error)"=w518) -> ("error out"=w534:errorcluster)  [unwired: 13 in]
      }
      frame "/**********MULTIPLE MIGRATION**********/" {
      }
      frame "Update Measurement Paths" {
        w570 = 70  # Remaining Progress
        # "Update the measurement file paths for measurement folder"
        n231 = property on="Progress" class="Slide (strict)"(error in=w560, "Value"=5 ("Progress"), "Caption.Text"="Getting paths...") -> (error out=w571:errorcluster)  [unwired: 1 in, 1 out]
        n232 = Unbundle By Name(w576) -> ("Migration Status"=w564:string[][], "Measurement Plug-ins"=w566:string[][], "Measurement file/folder path"=w579:path, "Measurement Plug-ins"=w578:string[][], "Measurement folder selected?"=w577:bool)
        n233 = property on="Measurement Count" class="Slide (strict)"(error in=w571, "Value"=0 ("Measurement Count"), "Caption.Text"="Updating Measurement Paths") -> (error out=w567:errorcluster)  [unwired: 1 in, 1 out]
        n234 = Index Array(array=w566, index (col)=1 ("disabled index (col)")) -> (element=w562:string[])  [unwired: 1 in]
        n235 = call "Get Measurement Paths.vi"("Measurement Path"=w579, "Measurement Plug-ins"=w578, "Measurement folder selected?"=w577, "error in"=w567) -> ("Measurement Path Array"=w574:path[], "error out"=w556:errorcluster)  [unwired: 10 in]
        n236 = Insert Into Array(array=w564, index (col)=0 ("disabled index (col)"), new element=w562) -> (w561:string[][])  [unwired: 1 in]
        n237 = Array Size(array=w574) -> (size(s)=w569:i32)
        n238 = Quotient & Remainder(x=w570, y=w569) -> (floor(x/y)=w568:i32)  [unwired: 1 out]
        n239 = Bundle By Name(cluster=w576, "Migration Status"=w561, "Measurement File Paths"=w574, "Plugin Migration Value"=w569, "Progress per measurement"=w568) -> (w575:T3)
        n240 = property on="Progress" class="Slide (strict)"(error in=w556, "Value"=15 ("Progress")) -> (error out=w555:errorcluster)  [unwired: 1 in, 1 out]
      }
      frame "Create Project" {
        # "Check if project exists and creates a new project if not present."
        n241 = property on="Progress" class="Slide (strict)"(error in=w583, "Value"=10 ("Progress"), "Caption.Text"="Checking for project...") -> (error out=w584:errorcluster)  [unwired: 1 in, 1 out]
        n242 = property on="Measurement Count" class="Slide (strict)"(error in=w584, "Value"=10 ("Measurement Count"), "Caption.Text"="Creating project if not exist") -> (error out=w587:errorcluster)  [unwired: 1 in, 1 out]
        n243 = Unbundle By Name(w591) -> ("Project path"=w590:path)
        n244 = call "Create and Save Project.vi"("Project Path"=w590, "error in (no error)"=w587) -> ("error out"=w581:errorcluster)  [unwired: 13 in]
        n245 = property on="Progress" class="Slide (strict)"(error in=w581, "Value"=15 ("Progress")) -> (error out=w580:errorcluster)  [unwired: 1 in, 1 out]
      }
      frame "Migrate measurements" {
        # "Migrate multiple measurements along with their shared dependencies"
        n246 = property on="Progress" class="Slide (strict)"(error in=w593, "Value"=0 ("Progress")) -> (error out=w594:errorcluster)  [unwired: 1 in, 1 out]
        n247 = Unbundle By Name(w604) -> ("Project path"=w608:path, "Measurement File Paths"=w606:path[], "Measurement Plug-ins"=w609:string[][])
        n248 = property on="Measurement Count" class="Slide (strict)"(error in=w594, "Value"=20 ("Measurement Count"), "Caption.Text"="Migrating measurement(s)") -> (error out=w599:errorcluster)  [unwired: 1 in, 1 out]
        n249 = Index Array(array=w609, index (col)=1 ("disabled index (col)")) -> (element=w607:string[])  [unwired: 1 in]
        n250 = control-ref of="Progress"() -> (w592:refnum<vi>)
        n251 = call "Migrate Dependencies.vi"("Project path"=w608, "Measurement paths"=w606, "Plug-in names"=w607, "Progress"=w592, "error in"=w599) -> ("Instrument containing subVIs"=w603:path[][], "error out"=w597:errorcluster)  [unwired: 9 in]
        n252 = Bundle By Name(cluster=w604, "Instrument containing subVIs"=w603, "Measurement Progress"=30) -> (w605:T3)
        n253 = property on="Measurement Count" class="Slide (strict)"(error in=w597, "Value"=30 ("Measurement Count")) -> (error out=w596:errorcluster)  [unwired: 1 in, 1 out]
      }
      frame "Enqueue Migration Steps" {
        # "Enqueue the set of states for measurement migration"
        n254 = Unbundle By Name(w615) -> ("Plugin Migration Value"=w614:i32)
        n255 = Greater Than 0?(x=w614) -> (x > 0?=w613:bool)
        n256 = case shown="True" w613 {
          tunnel: w612 -> [w618 w625]
          tunnel: [w620 w624] -> w611
          frame False {
            # "Enqueue next step if all measurements are migrated"
            n257 = property on="Measurement Count" class="Slide (strict)"(error in=w618, "Value"=100 ("Progress")) -> (error out=w619:errorcluster)  [unwired: 1 in, 1 out]
            n258 = call "Queue Driver.vi"("States[]"=string[] ["Save Project", "Show Next Steps"], "error in (no error)"=w619, "Q Operations"=Queue_Operations."Enqueue N") -> ("error out"=w620:errorcluster)  [unwired: 11 in, 1 out]
          }
          frame True {
            # "Enqueue, if there are measurements yet to migrate"
            n259 = call "Queue Driver.vi"("States[]"=string[] ["Set Values in Dict", "Create Plugin Template", "Get Driver List", "Edit Measurement Configuration", "Edit Measurement Results", "Edit Measurement Connector Pane", "Create Wrapper", "Deserialize Cluster Data", "Add Measurement Plugin APIs", "Disable Initialize APIs", "Edit Type Specialization", "Add UI Elements", "Flatten the Clusters", "Handling Default Value", "Update Migration Count"], "error in (no error)"=w625, "Q Operations"=Queue_Operations."Enqueue N") -> ("error out"=w624:errorcluster)  [unwired: 11 in, 1 out]
          }
        }
      }
      frame "Set Values in Dict" {
        # "Measurement Status Message: Migrating 1 of N measurement(s)"
        # "Set values to the Dictionary APIs"
        n260 = Unbundle By Name(w648) -> ("Project path"=w642:path, "Instrument containing subVIs"=w638:path[][], "Measurement Plug-ins"=w647:string[][], "Migration Count"=w626:i32, "Measurement File Paths"=w635:path[])
        n261 = property on="Progress" class="Slide (strict)"(error in=w629, "Value"=0 ("Progress")) -> (error out=w634:errorcluster)  [unwired: 1 in, 1 out]
        n262 = Array Size(array=w635) -> (size(s)=w627:i32)
        n263 = Increment(x=w626) -> (x+1=w631:i32)
        n264 = Format Into String(format string="Migrating %d of %d measurement(s)", error in=w634, w631, w627) -> (resulting string=w632:string, error out=w633:errorcluster)  [unwired: 1 in]
        n265 = property on="Measurement Count" class="Slide (strict)"(error in=w633, "Caption.Text"=w632) -> (error out=w636:errorcluster)  [unwired: 1 in, 1 out]
        n266 = Index Array(array=w635, index=w626) -> (element=w645:path)
        n267 = call "Set Code Module Path.vi"("CodeModule Path"=w645, "error in (no error)"=w636) -> ("error out"=w644:errorcluster)  [unwired: 13 in]
        n268 = Index Array(array=w647, index (row)=w626, index (col)=1 ("disabled index (col)")) -> (element=w643:string)
        n269 = Index Array(array=w638, index (row)=w626) -> (element=w641:path[])  [unwired: 1 in]
        n270 = call "Set Measurement Name.vi"("Name"=w643, "error in (no error)"=w644) -> ("error out"=w640:errorcluster)  [unwired: 13 in]
        n271 = call "Set Instrument VI Paths.vi"("error in (no error)"=w640, "VI Paths[]"=w641) -> ("error out"=w639:errorcluster)  [unwired: 9 in]
        n272 = call "Set Project Path.vi"("Project Path"=w642, "error in (no error)"=w639) -> ("error out"=w628:errorcluster)  [unwired: 13 in]
      }
      frame "Create Plugin Template" {
        # "Create Measurement Plugin Template"
        n273 = property on="Progress" class="Slide (strict)"(error in=w651, "Value"=1 ("Progress"), "Caption.Text"="Creating Measurement Plugin...") -> (error out=w652:errorcluster)  [unwired: 1 in, 1 out]
        n274 = Unbundle By Name(w656) -> ("Project path"=w655:path)
        n275 = call "Create Plugin Template.vi"("Project Path"=w655, "error in (no error)"=w652) -> ("error out"=w654:errorcluster)  [unwired: 13 in]
        n276 = call "Copy Set Default Value Multiple.vi"("error in (no error)"=w654) -> ("error out"=w650:errorcluster)  [unwired: 14 in]
      }
      frame "Get Driver List" {
        # "Get the list of instrument drivers used in the measurement"
        n277 = property on="Progress" class="Slide (strict)"(error in=w658, "Value"=3 ("Progress"), "Caption.Text"="Fetching the list of instrument drivers used...") -> (error out=w659:errorcluster)  [unwired: 1 in, 1 out]
        n278 = call "List Drivers.vi"("error in (no error)"=w659) -> ("error out"=w660:errorcluster)  [unwired: 14 in]
      }
      frame "Edit Measurement Configuration" {
        # "Add elements to the measurement configuration control file"
        n279 = property on="Progress" class="Slide (strict)"(error in=w664, "Value"=4 ("Progress"), "Caption.Text"="Editing measurement configuration...") -> (error out=w665:errorcluster)  [unwired: 1 in, 1 out]
        n280 = call "Add Measurement Plugin Controls.vi"("error in (no error)"=w665) -> ("error out"=w666:errorcluster)  [unwired: 14 in]
      }
      frame "Edit Measurement Results" {
        # "Add elements to the measurement results control file"
        n281 = property on="Progress" class="Slide (strict)"(error in=w670, "Value"=5 ("Progress"), "Caption.Text"="Editing measurement results...") -> (error out=w671:errorcluster)  [unwired: 1 in, 1 out]
        n282 = call "Add Meas Plugin Indicators.vi"("error in (no error)"=w671) -> ("error out"=w672:errorcluster)  [unwired: 14 in]
      }
      frame "Edit Measurement Connector Pane" {
        # "Edit the connector pane of the duplicated measurement"
        n283 = property on="Progress" class="Slide (strict)"(error in=w676, "Value"=6 ("Progress"), "Caption.Text"="Editing the connector pane of the measurement...") -> (error out=w677:errorcluster)  [unwired: 1 in, 1 out]
        n284 = call "Edit Connector Pane Multiple.vi"("error in (no error)"=w677) -> ("error out"=w678:errorcluster)  [unwired: 14 in]
      }
      frame "Create Wrapper" {
        # "Create a wrapper for the measurement"
        n285 = property on="Progress" class="Slide (strict)"(error in=w682, "Value"=7 ("Progress"), "Caption.Text"="Creating wrapper for the measurement...") -> (error out=w683:errorcluster)  [unwired: 1 in, 1 out]
        n286 = call "Create Wrapper for Measurement Plugin.vi"("error in (no error)"=w683) -> ("error out"=w684:errorcluster)  [unwired: 14 in]
      }
      frame "Deserialize Cluster Data" {
        # "Deserialize the connection in the wrapper vi"
        n287 = property on="Progress" class="Slide (strict)"(error in=w688, "Value"=8 ("Progress"), "Caption.Text"="Flattening and unflattening the cluster data in Wrapper...") -> (error out=w689:errorcluster)  [unwired: 1 in, 1 out]
        n288 = call "Deserialize Connections in Wrapper Plugin.vi"("error in (no error)"=w689) -> ("error out"=w690:errorcluster)  [unwired: 14 in]
      }
      frame "Add Measurement Plugin APIs" {
        # "Add all the rquired Measurement Plugin APIs in measurement logic and wire them appropriately"
        n289 = property on="Progress" class="Slide (strict)"(error in=w694, "Value"=9 ("Progress"), "Caption.Text"="Editing measurement logic...") -> (error out=w695:errorcluster)  [unwired: 1 in, 1 out]
        n290 = call "Create Measurement Plugin subVIs.vi"("error in (no error)"=w695) -> ("error out"=w696:errorcluster)  [unwired: 14 in]
      }
      frame "Disable Initialize APIs" {
        # "Disable the initialize and close in the measurement"
        n291 = property on="Progress" class="Slide (strict)"(error in=w700, "Value"=10 ("Progress"), "Caption.Text"="Disabling and removing the Initalize and Close APIs...") -> (error out=w701:errorcluster)  [unwired: 1 in, 1 out]
        n292 = call "Add Diagram disable structure.vi"("error in (no error)"=w701) -> ("error out"=w702:errorcluster)  [unwired: 14 in]
      }
      frame "Edit Type Specialization" {
        # "Edit the Type Specializations.vi"
        n293 = property on="Progress" class="Slide (strict)"(error in=w706, "Value"=11 ("Progress"), "Caption.Text"="Editing the Type Specialization VI...") -> (error out=w707:errorcluster)  [unwired: 1 in, 1 out]
        n294 = call "Edit Plugin Type Specialization.vi"("error in (no error)"=w707) -> ("error out"=w708:errorcluster)  [unwired: 14 in]
      }
      frame "Add UI Elements" {
        # "Edit the Measurement UI.vi"
        n295 = property on="Progress" class="Slide (strict)"(error in=w712, "Value"=12 ("Progress"), "Caption.Text"="Editing Measurement UI...") -> (error out=w713:errorcluster)  [unwired: 1 in, 1 out]
        n296 = call "Add Elements to Meas Plugin UI.vi"("error in (no error)"=w713) -> ("error out"=w714:errorcluster)  [unwired: 14 in]
      }
      frame "Flatten the Clusters" {
        # "Creating string ande serialize data for the wrapper connections"
        n297 = property on="Progress" class="Slide (strict)"(error in=w718, "Value"=13 ("Progress"), "Caption.Text"="Creating events and flatten the data...") -> (error out=w719:errorcluster)  [unwired: 1 in, 1 out]
        n298 = call "Create String and Serialize Cluster Data in UI.vi"("error in (no error)"=w719) -> ("error out"=w720:errorcluster)  [unwired: 14 in]
      }
      frame "Handling Default Value" {
        # "Setting default value for cluster based on string controls"
        n299 = property on="Progress" class="Slide (strict)"(error in=w724, "Value"=14 ("Progress"), "Caption.Text"="Loading values for string controls in UI...") -> (error out=w725:errorcluster)  [unwired: 1 in, 1 out]
        n300 = call "Logic for Default Case Multiple.vi"("error in (no error)"=w725) -> ("error out"=w726:errorcluster)  [unwired: 14 in]
      }
      frame "Save Project" {
        # "Saving the project and libraries"
        n301 = property on="Progress" class="Slide (strict)"(error in=w730, "Value"=15 ("Progress"), "Caption.Text"="Saving the project files...") -> (error out=w732:errorcluster)  [unwired: 1 in, 1 out]
        n302 = call "Save Projects and Libraries.vi"("error in (no error)"=w732) -> ("error out"=w731:errorcluster)  [unwired: 10 in]
      }
      frame "Update Migration Count" {
        # "Updating the migration count and migration status"
        n303 = in-place {
          in-place-border: [w743] -> w737
          n304 = in-place-cluster #2(w742) -> ("Plugin Migration Value"=w755:i32, "Migration Count"=w746:i32, "Measurement Progress"=w753:i32, "Progress per measurement"=w752:i32, "Migration Status"=w749:string[][])
          n305 = Index Array(array=w749, index (col)=1 ("disabled index (col)")) -> (element=w747:string[])  [unwired: 1 in]
          n306 = Insert Into Array(array=w747, index=w746, new element="Success") -> (w744:string[])
          n307 = Insert Into Array(array=w749, index (col)=1 ("disabled index (col)"), new element=w744) -> (w751:string[][])  [unwired: 1 in]
          n308 = Increment(x=w746) -> (x+1=w756:i32)
          n309 = Add(x=w753, y=w752) -> (x+y=w743:i32)
          n310 = Decrement(x=w755) -> (x-1=w754:i32)
          n311 = in-place-cluster #2("Plugin Migration Value"=w754, "Migration Count"=w756, "Measurement Progress"=w743, "Progress per measurement"=w752, "Migration Status"=w751) -> (w741:T3)
        }
        n312 = property on="Measurement Count" class="Slide (strict)"(error in=w736, "Value"=w737) -> (error out=w735:errorcluster)  [unwired: 1 in, 1 out]
        n313 = call "Queue Driver.vi"("State"="Enqueue Migration Steps", "error in (no error)"=w735, "Q Operations"=Queue_Operations."Enqueue") -> ("error out"=w740:errorcluster)  [unwired: 11 in, 1 out]
      }
      frame "Update count on Fail" {
        # "Updating the migration count and migration status"
        n314 = in-place {
          in-place-border: [w765] -> w759
          n315 = in-place-cluster #3(w764) -> ("Plugin Migration Value"=w777:i32, "Migration Count"=w768:i32, "Measurement Progress"=w775:i32, "Progress per measurement"=w774:i32, "Migration Status"=w771:string[][])
          n316 = Index Array(array=w771, index (col)=1 ("disabled index (col)")) -> (element=w769:string[])  [unwired: 1 in]
          n317 = Insert Into Array(array=w769, index=w768, new element="Fail") -> (w766:string[])
          n318 = Insert Into Array(array=w771, index (col)=1 ("disabled index (col)"), new element=w766) -> (w773:string[][])  [unwired: 1 in]
          n319 = Increment(x=w768) -> (x+1=w778:i32)
          n320 = Add(x=w775, y=w774) -> (x+y=w765:i32)
          n321 = Decrement(x=w777) -> (x-1=w776:i32)
          n322 = in-place-cluster #3("Plugin Migration Value"=w776, "Migration Count"=w778, "Measurement Progress"=w765, "Progress per measurement"=w774, "Migration Status"=w773) -> (w763:T3)
        }
        n323 = property on="Measurement Count" class="Slide (strict)"(error in=w758, "Value"=w759) -> (error out=w757:errorcluster)  [unwired: 1 in, 1 out]
        n324 = call "Queue Driver.vi"("State"="Enqueue Migration Steps", "error in (no error)"=w757, "Q Operations"=Queue_Operations."Enqueue") -> ("error out"=w762:errorcluster)  [unwired: 11 in, 1 out]
      }
      frame "/**********NEXT STEPS POST MIGRATION**********/" {
      }
      frame "Show Next Steps" {
        # "To change unwanted loading symbol"
        # "Showing the migration status"
        n325 = in-place {
          in-place-border: [w804] -> w788
          n326 = in-place-cluster #4(w796) -> ("Migration Status"=w805:string[][])
          n327 = Index Array(array=w805, index (col) #1=0 ("disabled index (col)"), index (col) #2=1 ("index (col)")) -> (element #1=w808:string[], element #2=w806:string[])  [unwired: 2 in]
          n328 = for {
            tunnel: w808 -> [_] mode=indexing
            tunnel: w806 -> [w815]
            shift-right: [w810] -> w804
            shift-left: w805 -> [w813]
            i -> [w812]
            n329 = Index Array(array=w815, index=w812) -> (element=w814:string)
            n330 = Empty String/Path?(string/path=w814) -> (empty?=w811:bool)
            n331 = case shown="True" w811 {
              tunnel: w813 -> [w816 w823]
              tunnel: w812 -> [_ w820]
              tunnel: [w816 w824] -> w810
              frame False {
              }
              frame True {
                # "Insert 'Fail' for empty status"
                n332 = Index Array(array=w823, index (col)=1 ("disabled index (col)")) -> (element=w821:string[])  [unwired: 1 in]
                n333 = Insert Into Array(array=w821, index=w820, new element="Fail" ("new element/subarray")) -> (w818:string[])
                n334 = Insert Into Array(array=w823, index (col)=1 ("disabled index (col)"), new element=w818) -> (w824:string[][])  [unwired: 1 in]
              }
            }
          }
          n335 = in-place-cluster #4("Migration Status"=w804) -> (w795:T3)
        }
        n336 = property on="Tab Control" class="TabCtl (strict)"(error in=w791, "Value"=T1."Status" ("Tab Control")) -> (error out=w793:errorcluster)  [unwired: 1 in, 1 out]
        n337 = property on="Migration Status" class="MCListbox (strict)"(error in=w793, "Allow Editing Cells"=FALSE) -> (error out=w792:errorcluster)  [unwired: 1 in, 1 out]
        n338 = property on="Migration Status" class="MCListbox (strict)"(error in=w792, "ItemNames"=w788) -> (error out=w783:errorcluster)  [unwired: 1 in, 1 out]
        n339 = Index Array(array=w788, index (col)=1 ("disabled index (col)")) -> (element=w786:string[])  [unwired: 1 in]
        n340 = Equal?(x=w786, y="Fail" ("new element/subarray")) -> (x = y?=w784:bool[])
        n341 = And Array Elements(Boolean array=w784) -> (logical AND=w781:bool)
        n342 = case "All the measurements failed?" shown="True" w781 {
          tunnel: w783 -> [w799 w803]
          tunnel: [w800 w802] -> w782
          frame False {
            n343 = property on="Review" class="Bool"(error in=w799, "BoolText.Text"="Review Plug-ins" ("Boolean Text.Text")) -> (error out=w800:errorcluster)  [unwired: 1 in, 1 out]
          }
          frame True {
            # "Change Bool Text to Start next migration"
            n344 = property on="Review" class="Bool"(error in=w803, "BoolText.Text"="Start Next Migration" ("Boolean Text.Text")) -> (error out=w802:errorcluster)  [unwired: 1 in, 1 out]
          }
        }
        n345 = call "Set Cursor Icon.vi"("Cursor icon"=u16 0, "error in (no error)"=w782) -> ("error out"=w790:errorcluster)  [unwired: 13 in]
      }
      frame "Show Links" {
        # "Showing links for the migrated measurements"
        n346 = Unbundle By Name(w832) -> ("Migration Status"=w834:string[][])
        n347 = for {
          tunnel: w834 -> [w841] mode=indexing
          tunnel: [w835] -> w829 mode=indexing if=w838
          # "Populating combo box with successfully migrated plugin names"
          n348 = Index Array(array=w841, index #1=0 ("index"), index #2=1 ("index")) -> (element #1=w835:string, element #2=w836:string)
          n349 = Equal?(x=w836, y="Success") -> (x = y?=w838:bool)
        }
        n350 = Index Array(array=w829, index=0) -> (element=w825:string)
        n351 = property on="Select Plug-in" class="CmbBox"(error in=w833, "Strings[]"=w829, "Value"=w825) -> (error out=w827:errorcluster)  [unwired: 1 in, 1 out]
        n352 = call "Set Measurement Name.vi"("Name"=w825, "error in (no error)"=w827) -> ("error out"=w826:errorcluster)  [unwired: 13 in]
        n353 = property on="Tab Control" class="TabCtl (strict)"(error in=w826, "Value"=T1."Links" ("Tab Control")) -> (error out=w830:errorcluster)  [unwired: 1 in, 1 out]
      }
      frame "/**********ERROR**********/" {
      }
      frame "Error" {
        # "Handle the error and alert user"
        n354 = call <vilib>:"Clear Errors.vi"("error in (no error)"=w851) -> ("error out"=w852:errorcluster)  [unwired: 5 in, 1 out]
        n355 = Equal?(x=string[] ["Set Values in Dict", "Create Plugin Template", "Get Driver List", "Edit Measurement Configuration", "Edit Measurement Results", "Edit Measurement Connector Pane", "Create Wrapper", "Deserialize Cluster Data", "Add Measurement Plugin APIs", "Disable Initialize APIs", "Edit Type Specialization", "Add UI Elements", "Flatten the Clusters", "Handling Default Value", "Update Migration Count"] ("States[]"), y=w844) -> (x = y?=w846:bool[])
        n356 = call "Queue Driver.vi"("error in (no error)"=w852, "Q Operations"=Queue_Operations."Flush") -> ("error out"=w849:errorcluster)  [unwired: 12 in, 1 out]
        n357 = Or Array Elements(Boolean array=w846) -> (logical OR=w845:bool)
        n358 = case shown="True" w845 {
          tunnel: w849 -> [w859 w871]
          tunnel: [w858 w869] -> w848
          tunnel: w844 -> [w857 _]
          frame False {
            # "If error occurs in other steps"
            n359 = Equal?(x=string[] ["Update Measurement Paths", "Create Project", "Migrate measurements"] ("States[]"), y=w857) -> (x = y?=w855:bool[])
            n360 = Or Array Elements(Boolean array=w855) -> (logical OR=w854:bool)
            n361 = case "Error in Migration?" shown="False" w854 {
              tunnel: w859 -> [w863 w866]
              tunnel: [w862 w865] -> w858
              frame False {
                # "Restart Migration tool"
                n362 = call "Queue Driver.vi"("States[]"=string[] ["Reinitialize", "Initialize UI", "Populate project path"], "error in (no error)"=w863, "Q Operations"=Queue_Operations."Enqueue N") -> ("error out"=w862:errorcluster)  [unwired: 11 in, 1 out]
              }
              frame True {
                # "Show Next steps"
                n363 = call "Queue Driver.vi"("State"="Show Next Steps", "error in (no error)"=w866, "Q Operations"=Queue_Operations."Enqueue") -> ("error out"=w865:errorcluster)  [unwired: 11 in, 1 out]
              }
            }
          }
          frame True {
            # "If error occurs during measurement migration"
            n364 = call "Queue Driver.vi"("State"="Update count on Fail", "error in (no error)"=w871, "Q Operations"=Queue_Operations."Enqueue") -> ("error out"=w869:errorcluster)  [unwired: 11 in, 1 out]
          }
        }
      }
      frame "/**********EXIT**********/" {
      }
      frame "Exit" {
        # "Flush the queue elements and stop execution"
        n365 = call "Queue Driver.vi"("error in (no error)"=w884, "Q Operations"=Queue_Operations."Flush") -> ("error out"=w878:errorcluster)  [unwired: 12 in, 1 out]
        n366 = call "Queue Driver.vi"("error in (no error)"=w878, "Q Operations"=Queue_Operations."Release") -> ("error out"=w877:errorcluster)  [unwired: 12 in, 1 out]
        n367 = Unbundle By Name(w882) -> ("Tree Reference"=w881:refnum<vi>)
        n368 = Close Reference(reference=w881, error in (no error)=w877) -> (error out=w875:errorcluster)
        n369 = call "Dictionary.vi"("error in (no error)"=w875, "Dict States"=Dictionary_States."Delete All") -> ("error out"=w874:errorcluster)  [unwired: 12 in, 1 out]
      }
    }
  }
  n370 = invoke class="VI" method="FP.Close"(error in=w6) -> (error out=→"error out":errorcluster)  [unwired: 2 in, 2 out]
